vi "氨氮总磷平行样流程.vi"(9 "总磷1":bool, 10 "氨氮1":bool, 11 "队列输入":refnum<queue>) -> (3 "布尔":bool)   [LabVIEW 2016, in "质控单元.lvlib"]
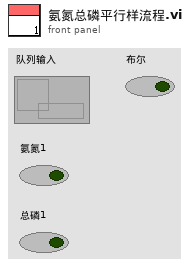
[diagram p1: front panel]
types:
  T1 = enum16{"待机", "启动氨氮水样", "氨氮测量中", "启动氨氮加标", "启动氨氮加标回收", "氨氮加标回收测量中", "启动总磷水样", "总磷水样测量中", "启动总磷加标", "启动总磷加标回收", "总磷加标回收测量中", "结束"}
  T2 = cluster{"站号":u16, "量程切换":enum32{"H", "L", "AUTO"}, "控制命令":enum16{"启动测量", "标样核查", "零点核查", "跨度核查", "空白测试", "平行样测试", "加标回收", "空白校准", "标样校准", "初始化（清洗）", "停止测试", "仪器重启", "校时", "模式设置", "测量间隔设置", "盲样测试"}, "模式设置":enum16{"待机", "连续模式", "周期模式", "定点模式", "受控模式", "手动模式"}, "测量间隔":u16}
  T3 = cluster{"时间标识":timestamp, "设备":string, "日志信息":string}
  T4 = cluster{"系统时间":timestamp, "工作状态":enum16{"空闲", "水样测试", "标样核查", "零点核查", "跨度核查", "空白测试", "平行样测试", "加标回收", "空白校准", "标样校准", "初始化（清洗）"}, "测量模式":enum16{"待机", "连续模式", "周期模式", "定点模式", "受控模式", "手动模式"}, "告警代码":u16, "故障代码":u16, "日志代码":u16, "软件版本":u16, "F0":sgl, "F1":sgl, "F2":sgl, "F3":sgl, "T":sgl, "H":sgl, "id":u16, "flowid":u16, "量程":u16, "总磷控温温度1":sgl, "营养盐控温温度2":sgl, "ADC":sgl}
  T5 = enum16{"空闲", "水样测试", "标样核查", "零点核查", "跨度核查", "空白测试", "平行样测试", "加标回收", "空白校准", "标样校准", "初始化（清洗）"}
  T6 = cluster{"因子编码":u32, "单位":u16, "标样参考值":sgl, "水样数据时间":timestamp, "水样实测值":sgl, "水样数据标识":string, "标样数据时间":timestamp, "标样实测值":sgl, "标样数据标识":string, "空白数据时间":timestamp, "空白实测值":sgl, "空白数据标识":string, "零点核查数据时间":timestamp, "零点核查实测值":sgl, "零点核查数据标识":string, "跨度核查数据时间":timestamp, "跨度核查实测值":sgl, "跨度核查数据标识":string, "加标回收数据时间":timestamp, "加标回收实测值":sgl, "加标回收数据标识":string, "平行样数据时间":timestamp, "平行样实测值":sgl, "平行样数据标识":string, "F0":sgl, "F1":sgl, "F2":sgl, "F3":sgl, "F4":sgl, "F5":sgl, "F6":sgl, "F7":sgl, "温度":sgl, "湿度":sgl, "X值":sgl, "fidrange":u16}
  T7 = cluster{"量程":dbl, "检出限":dbl, "加标前水样浓度":dbl, "加标后水样浓度":dbl, "加标水杯定容体积":dbl, "加标母液浓度":dbl, "加标体积":dbl, "加标回收率":dbl}
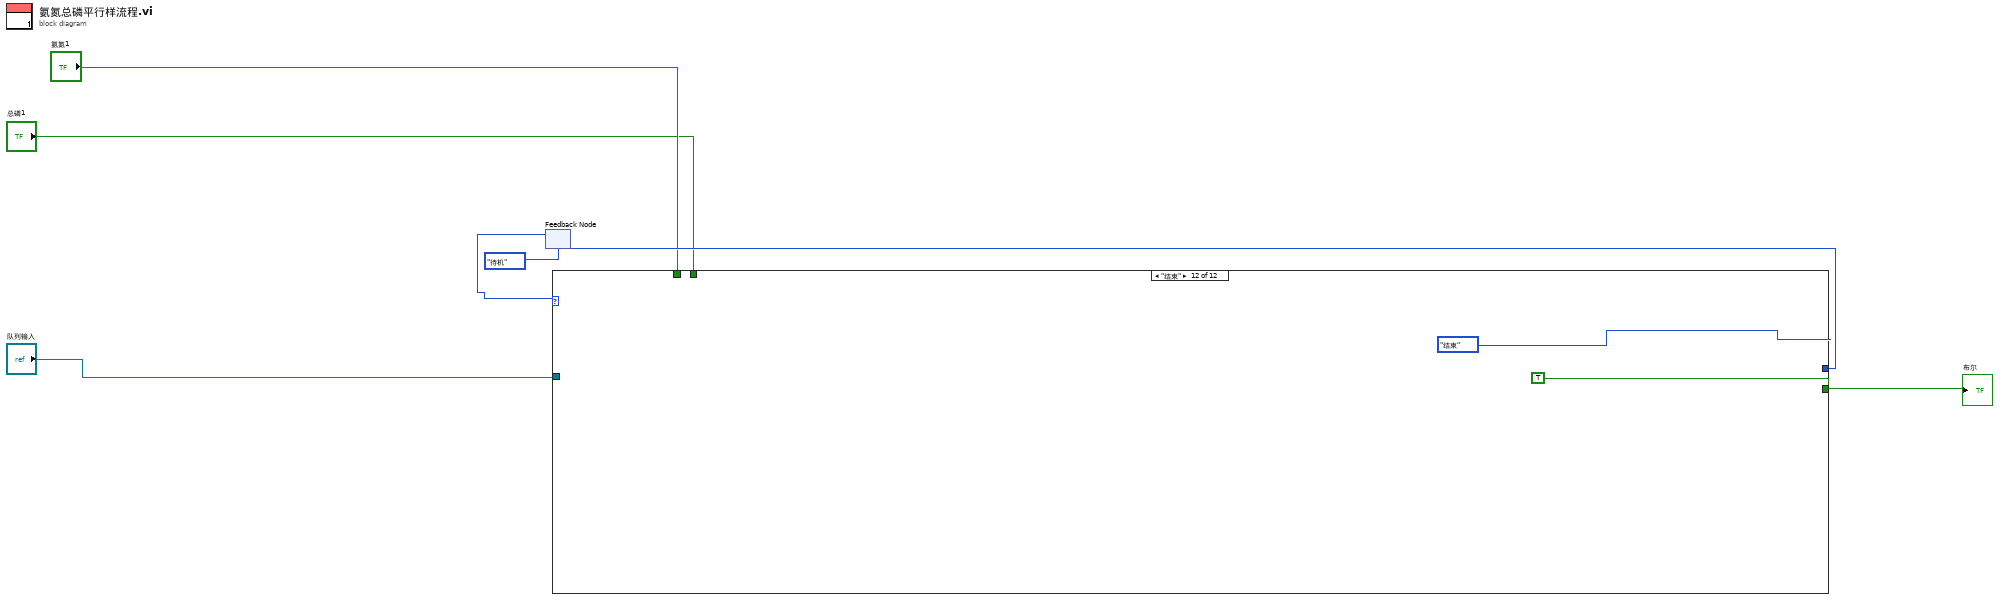
[diagram p0: block diagram]
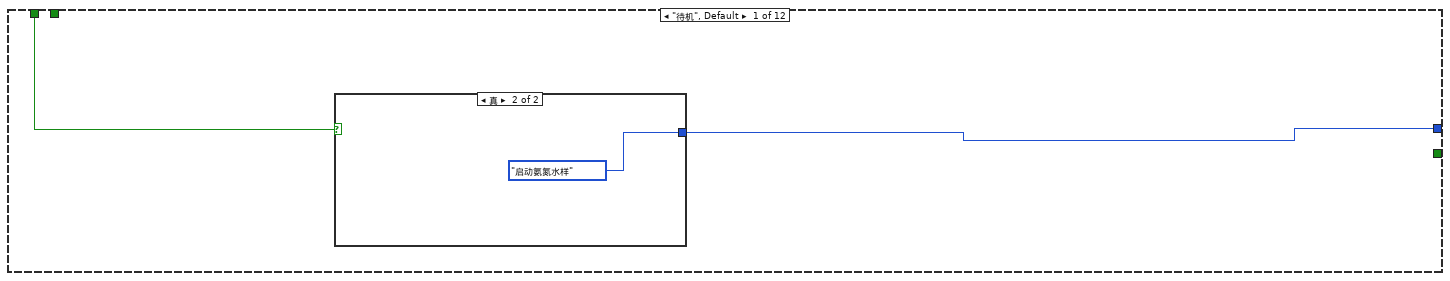
[diagram p2: hidden frame]
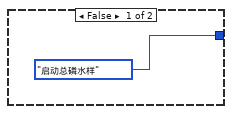
[diagram p3: hidden frame]
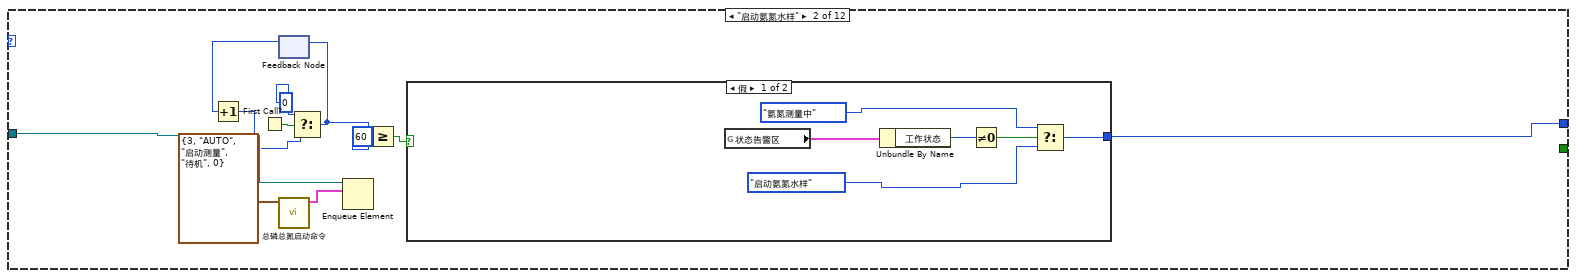
[diagram p4: hidden frame]
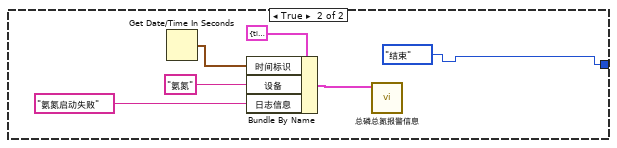
[diagram p5: hidden frame]
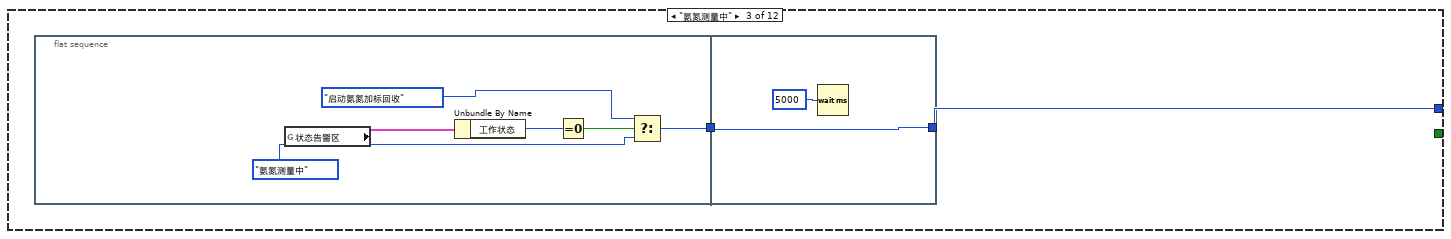
[diagram p6: hidden frame]
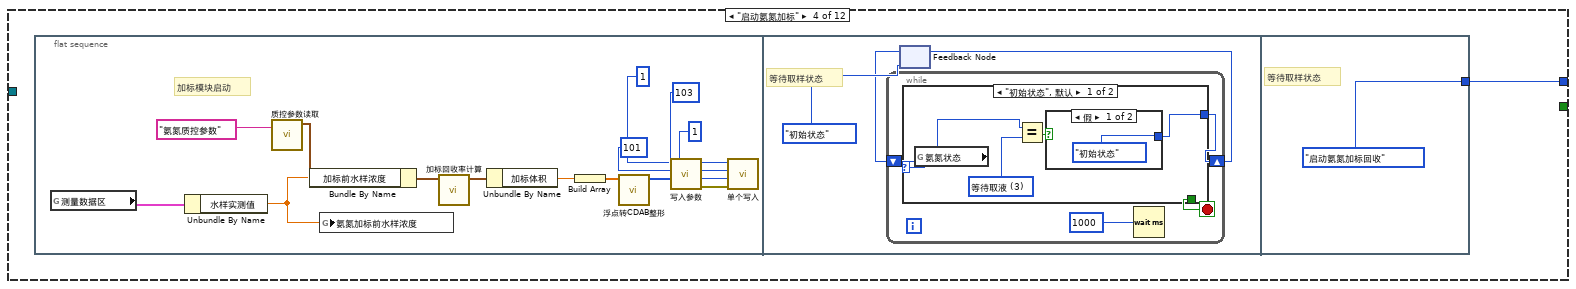
[diagram p7: hidden frame]
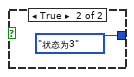
[diagram p8: hidden frame]
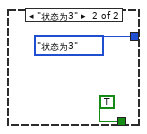
[diagram p9: hidden frame]
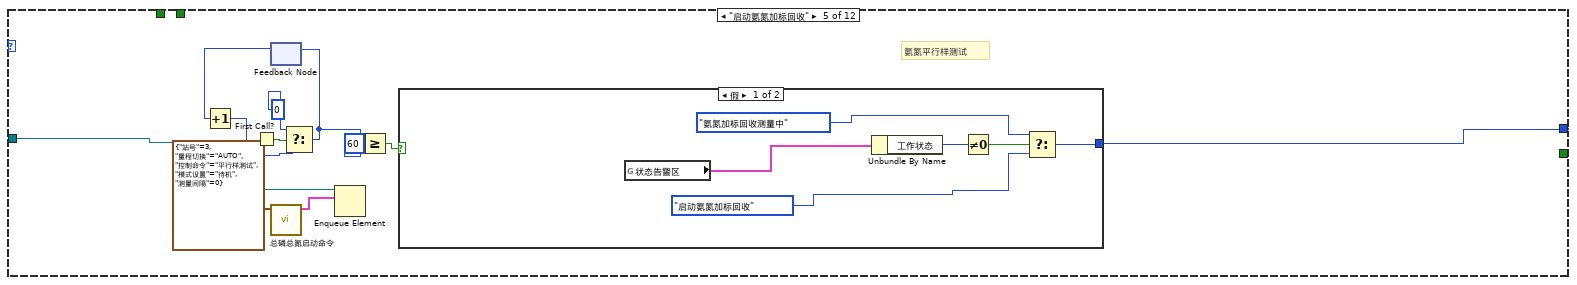
[diagram p10: hidden frame]
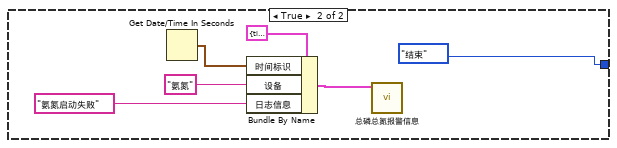
[diagram p11: hidden frame]
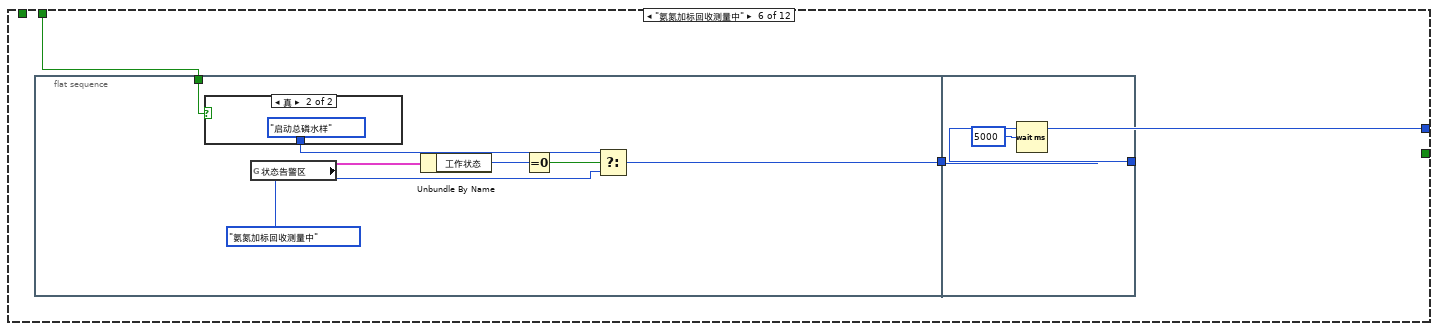
[diagram p12: hidden frame]
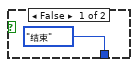
[diagram p13: hidden frame]
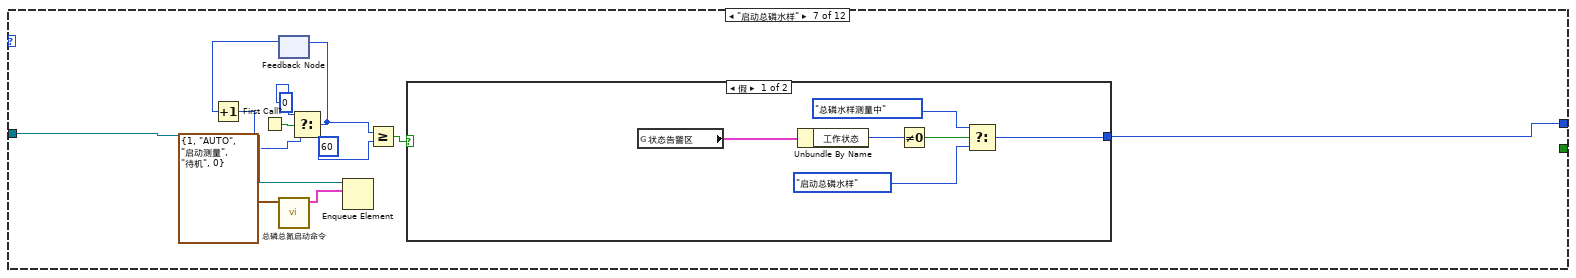
[diagram p14: hidden frame]
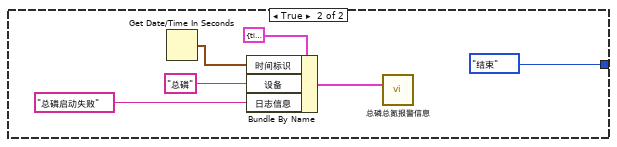
[diagram p15: hidden frame]
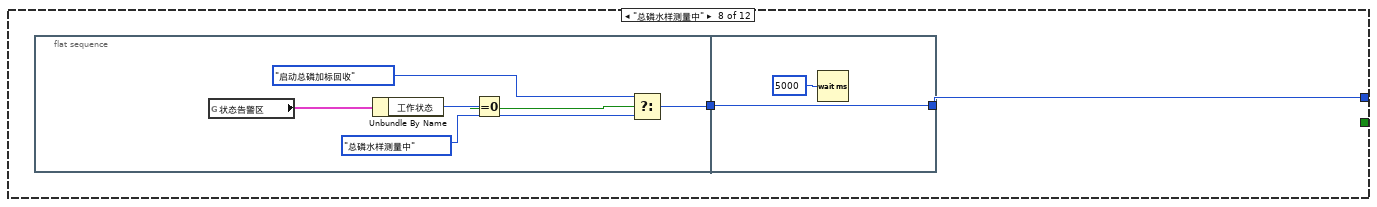
[diagram p16: hidden frame]
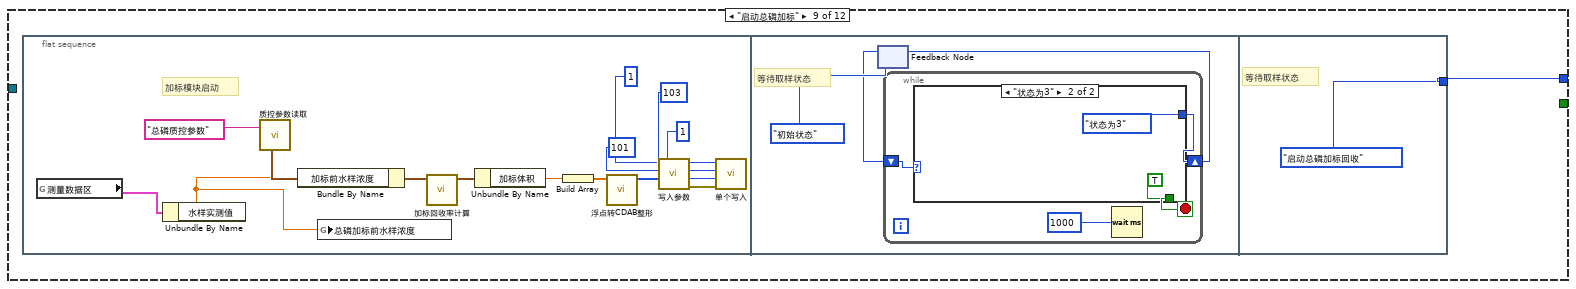
[diagram p17: hidden frame]
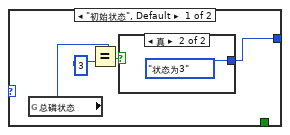
[diagram p18: hidden frame]
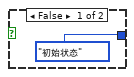
[diagram p19: hidden frame]
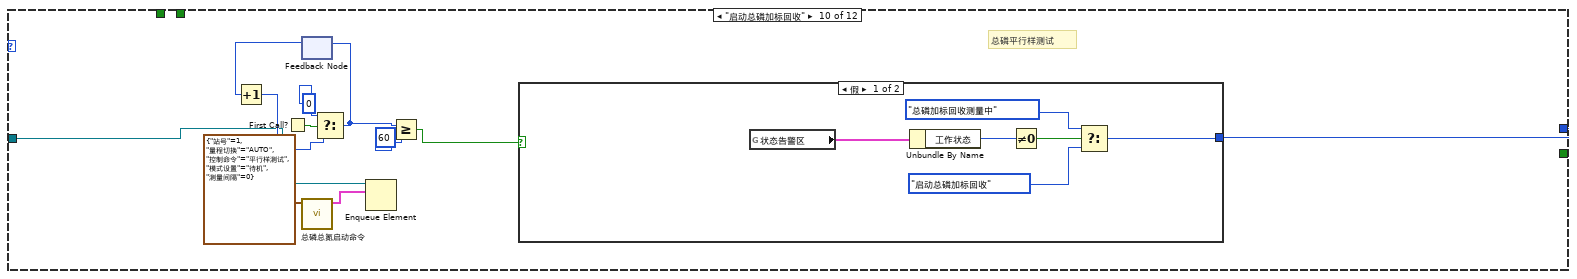
[diagram p20: hidden frame]
diagram:
  n1 = feedback #1(T1."待机") -> (w6:T1)
  n2 = case shown="\"结束\"" w6 {
    tunnel: [w8 w21 w36 w45 w76 w100 w122 w137 w146 w177 w200 T1."结束"] -> w5
    tunnel: "队列输入" -> [_ w22 _ _ w77 _ w123 _ _ w178 _ _]
    tunnel: [_ _ _ _ _ _ _ _ _ _ _ TRUE] -> w2
    tunnel: "总磷1" -> [_ _ _ _ _ w99 _ _ _ _ _ _]
    tunnel: "氨氮1" -> [w9 _ _ _ _ _ _ _ _ _ _ _]
    frame "待机", Default {
      n3 = case shown="真" w9 {
        tunnel: [T1."启动总磷水样" T1."启动氨氮水样"] -> w8
        frame False {
        }
        frame True {
        }
      }
    }
    frame "启动氨氮水样" {
      n4 = First Call?() -> (First Call?: T/F=w19:bool)
      n5 = feedback #2() -> (w18:i32)  [unwired: 1 in]
      n6 = Increment(x=w18) -> (x+1=w17:i32)
      n7 = call "总磷总氮启动命令.vi"("参数"=T2 {"站号"=3, "量程切换"=enum."AUTO", "控制命令"=enum."启动测量", "模式设置"=enum."待机", "测量间隔"=0}) -> ("启动命令"=w13:cluster{"命令":string, "data":variant})  [unwired: 10 in]
      n8 = Select(t=0, s=w19, f=w17) -> (s? t:f=w16:i32)
      n9 = feedback-in #2(w16) -> ()
      n10 = Enqueue Element(queue=w22, element=w13) -> ()  [unwired: 2 in, 3 out]
      n11 = Greater Or Equal?(x=w16, y=60) -> (x >= y?=w14:bool)
      n12 = case shown="假" w14 {
        tunnel: [w25 T1."结束"] -> w21
        frame False {
          n13 = global read "VAR总磷总氮全局变量.vi" "状态告警区"() -> (w28:T4)
          n14 = Unbundle By Name(w28) -> ("工作状态"=w27:T5)
          n15 = Not Equal To 0?(x=w27) -> (x != 0?=w26:bool)
          n16 = Select(t=T1."氨氮测量中", s=w26, f=T1."启动氨氮水样") -> (s? t:f=w25:T1)
        }
        frame True {
          n17 = Get Date/Time In Seconds() -> (seconds since 1Jan1904=w34:timestamp)
          n18 = Bundle By Name(cluster=T3 {"时间标识"=timestamp(0 s since 1904-01-01), "设备"="", "日志信息"=""} ("data in"), "时间标识"=w34, "设备"="氨氮", "日志信息"="氨氮启动失败") -> (w30:T3)
          n19 = call "总磷总氮报警信息.vi"("data in"=w30) -> ()  [unwired: 10 in, 1 out]
        }
      }
    }
    frame "氨氮测量中" {
      n20 = flat-sequence {
        tunnel: [w40] -> w35
        tunnel: [w44] -> w36
        tunnel: w35 -> [w44]
        frame #0 {
          n21 = global read "VAR总磷总氮全局变量.vi" "状态告警区"() -> (w41:T4)
          n22 = Unbundle By Name(w41) -> ("工作状态"=w42:T5)
          n23 = Equal To 0?(x=w42) -> (x = 0?=w39:bool)
          n24 = Select(t=T1."启动氨氮加标回收", s=w39, f=T1."氨氮测量中") -> (s? t:f=w40:T1)
        }
        frame #1 {
          n25 = Wait (ms)(milliseconds to wait=u32 5000 ("等待时间（毫秒）")) -> ()  [unwired: 1 out]
        }
      }
    }
    frame "启动氨氮加标" {
      n26 = flat-sequence {
        tunnel: [T1."启动氨氮加标回收"] -> w45
        frame #0 {
          w49 = u16 1 ("value")
          # "加标模块启动"
          n27 = global read "VAR总磷总氮全局变量.vi" "测量数据区"() -> (w47:T6)
          n28 = Unbundle By Name(w47) -> ("水样实测值"=w46:sgl)
          n29 = call "质控参数读取.vi"("section"="氨氮质控参数") -> ("参数"=w57:T7)  [unwired: 9 in, 1 out]
          n30 = Bundle By Name(cluster=w57, "加标前水样浓度"=w46) -> (w58:T7)
          n31 = global write "水样浓度全局.vi" "氨氮加标前水样浓度"(w46) -> ()
          n32 = call "加标回收率计算.vi"("参数"=w58) -> ("参数 out"=w56:T7)  [unwired: 10 in]
          n33 = Unbundle By Name(w56) -> ("加标体积"=w48:dbl)
          n34 = Build Array(w48) -> (w55:dbl[])
          n35 = call "浮点转CDAB整形.vi"("浮点数"=w55) -> ("CDAB整形输出"=w50:u16[])  [unwired: 10 in]
          n36 = call "写入参数.vi"("values"=w50, "starting address"=u16 101, "Slave ID"=w49) -> ("error out"=w54:errorcluster)  [unwired: 8 in]
          n37 = call "单个写入.vi"("Error in"=w54, "value"=u16 1, "address"=u16 103, "Slave ID"=w49) -> ()  [unwired: 7 in, 1 out]
        }
        frame #1 {
          # "等待取样状态"
          n38 = feedback #3(enum16{"初始状态", "状态为3"}."初始状态") -> (w61:enum16{"初始状态", "状态为3"})
          n39 = while {
            shift-right: [w65] -> w60
            shift-left: w61 -> [w66]
            stop <- w64 stop-if-true
            n40 = case shown="\"初始状态\", 默认" w66 {
              tunnel: [w68 enum16{"初始状态", "状态为3"}."状态为3"] -> w65
              tunnel: [_ TRUE] -> w64
              frame "初始状态", Default {
                w67 = u16 3 items=["待机", "润洗", "进样", "等待取液", "排液"] ("氨氮状态")
                n41 = global read "氨氮加标回收状态全局变量.vi" "氨氮状态"() -> (w70:u16)
                n42 = Equal?(x=w70, y=w67) -> (x = y?=w69:bool)
                n43 = case shown="假" w69 {
                  tunnel: [enum16{"初始状态", "状态为3"}."初始状态" enum16{"初始状态", "状态为3"}."状态为3"] -> w68
                  frame False {
                  }
                  frame True {
                  }
                }
              }
              frame "状态为3" {
              }
            }
            n44 = Wait (ms)(milliseconds to wait=u32 1000 ("等待时间（毫秒）")) -> ()  [unwired: 1 out]
          }
          n45 = feedback-in #3(w60) -> ()
        }
        frame #2 {
          # "等待取样状态"
        }
      }
    }
    frame "启动氨氮加标回收" {
      # "氨氮平行样测试"
      n46 = First Call?() -> (First Call?: T/F=w85:bool)
      n47 = feedback #4() -> (w84:i32)  [unwired: 1 in]
      n48 = Increment(x=w84) -> (x+1=w83:i32)
      n49 = call "总磷总氮启动命令.vi"("参数"=T2 {"站号"=3, "量程切换"=enum."AUTO", "控制命令"=enum."平行样测试", "模式设置"=enum."待机", "测量间隔"=0}) -> ("启动命令"=w79:cluster{"命令":string, "data":variant})  [unwired: 10 in]
      n50 = Select(t=0, s=w85, f=w83) -> (s? t:f=w82:i32)
      n51 = feedback-in #4(w82) -> ()
      n52 = Enqueue Element(queue=w77, element=w79) -> ()  [unwired: 2 in, 3 out]
      n53 = Greater Or Equal?(x=w82, y=60) -> (x >= y?=w80:bool)
      n54 = case shown="假" w80 {
        tunnel: [w89 T1."结束"] -> w76
        frame False {
          n55 = global read "VAR总磷总氮全局变量.vi" "状态告警区"() -> (w92:T4)
          n56 = Unbundle By Name(w92) -> ("工作状态"=w91:T5)
          n57 = Not Equal To 0?(x=w91) -> (x != 0?=w90:bool)
          n58 = Select(t=T1."氨氮加标回收测量中", s=w90, f=T1."启动氨氮加标回收") -> (s? t:f=w89:T1)
        }
        frame True {
          n59 = Get Date/Time In Seconds() -> (seconds since 1Jan1904=w98:timestamp)
          n60 = Bundle By Name(cluster=T3 {"时间标识"=timestamp(0 s since 1904-01-01), "设备"="", "日志信息"=""} ("data in"), "时间标识"=w98, "设备"="氨氮", "日志信息"="氨氮启动失败") -> (w94:T3)
          n61 = call "总磷总氮报警信息.vi"("data in"=w94) -> ()  [unwired: 10 in, 1 out]
        }
      }
    }
    frame "氨氮加标回收测量中" {
      n62 = flat-sequence {
        tunnel: [w106] -> w101
        tunnel: w99 -> [w102]
        tunnel: [w112] -> w100
        tunnel: w101 -> [w112]
        frame #0 {
          n63 = case shown="真" w102 {
            tunnel: [T1."结束" T1."启动总磷水样"] -> w104
            frame False {
            }
            frame True {
            }
          }
          n64 = global read "VAR总磷总氮全局变量.vi" "状态告警区"() -> (w107:T4)
          n65 = Unbundle By Name(w107) -> ("工作状态"=w108:T5)
          n66 = Equal To 0?(x=w108) -> (x = 0?=w103:bool)
          n67 = Select(t=w104, s=w103, f=T1."氨氮加标回收测量中") -> (s? t:f=w106:T1)
        }
        frame #1 {
          n68 = Wait (ms)(milliseconds to wait=u32 5000 ("等待时间（毫秒）")) -> ()  [unwired: 1 out]
        }
      }
    }
    frame "启动总磷水样" {
      n69 = First Call?() -> (First Call?: T/F=w120:bool)
      n70 = feedback #5() -> (w119:i32)  [unwired: 1 in]
      n71 = Increment(x=w119) -> (x+1=w118:i32)
      n72 = call "总磷总氮启动命令.vi"("参数"=T2 {"站号"=1, "量程切换"=enum."AUTO", "控制命令"=enum."启动测量", "模式设置"=enum."待机", "测量间隔"=0}) -> ("启动命令"=w114:cluster{"命令":string, "data":variant})  [unwired: 10 in]
      n73 = Select(t=0, s=w120, f=w118) -> (s? t:f=w117:i32)
      n74 = feedback-in #5(w117) -> ()
      n75 = Enqueue Element(queue=w123, element=w114) -> ()  [unwired: 2 in, 3 out]
      n76 = Greater Or Equal?(x=w117, y=60) -> (x >= y?=w115:bool)
      n77 = case shown="假" w115 {
        tunnel: [w126 T1."结束"] -> w122
        frame False {
          n78 = global read "VAR总磷总氮全局变量.vi" "状态告警区"() -> (w127:T4)
          n79 = Unbundle By Name(w127) -> ("工作状态"=w128:T5)
          n80 = Not Equal To 0?(x=w128) -> (x != 0?=w129:bool)
          n81 = Select(t=T1."总磷水样测量中", s=w129, f=T1."启动总磷水样") -> (s? t:f=w126:T1)
        }
        frame True {
          n82 = Get Date/Time In Seconds() -> (seconds since 1Jan1904=w135:timestamp)
          n83 = Bundle By Name(cluster=T3 {"时间标识"=timestamp(0 s since 1904-01-01), "设备"="", "日志信息"=""} ("data in"), "时间标识"=w135, "设备"="总磷", "日志信息"="总磷启动失败") -> (w131:T3)
          n84 = call "总磷总氮报警信息.vi"("data in"=w131) -> ()  [unwired: 10 in, 1 out]
        }
      }
    }
    frame "总磷水样测量中" {
      n85 = flat-sequence {
        tunnel: [w141] -> w136
        tunnel: [w145] -> w137
        tunnel: w136 -> [w145]
        frame #0 {
          n86 = global read "VAR总磷总氮全局变量.vi" "状态告警区"() -> (w142:T4)
          n87 = Unbundle By Name(w142) -> ("工作状态"=w143:T5)
          n88 = Equal To 0?(x=w143) -> (x = 0?=w140:bool)
          n89 = Select(t=T1."启动总磷加标回收", s=w140, f=T1."总磷水样测量中") -> (s? t:f=w141:T1)
        }
        frame #1 {
          n90 = Wait (ms)(milliseconds to wait=u32 5000 ("等待时间（毫秒）")) -> ()  [unwired: 1 out]
        }
      }
    }
    frame "启动总磷加标" {
      n91 = flat-sequence {
        tunnel: [T1."启动总磷加标回收"] -> w146
        frame #0 {
          w151 = u16 1 ("value")
          # "加标模块启动"
          n92 = global read "VAR总磷总氮全局变量.vi" "测量数据区"() -> (w149:T6)
          n93 = Unbundle By Name(w149) -> ("水样实测值"=w147:sgl)
          n94 = call "质控参数读取.vi"("section"="总磷质控参数") -> ("参数"=w148:T7)  [unwired: 9 in, 1 out]
          n95 = Bundle By Name(cluster=w148, "加标前水样浓度"=w147) -> (w159:T7)
          n96 = global write "水样浓度全局.vi" "总磷加标前水样浓度"(w147) -> ()
          n97 = call "加标回收率计算.vi"("参数"=w159) -> ("参数 out"=w158:T7)  [unwired: 10 in]
          n98 = Unbundle By Name(w158) -> ("加标体积"=w150:dbl)
          n99 = Build Array(w150) -> (w157:dbl[])
          n100 = call "浮点转CDAB整形.vi"("浮点数"=w157) -> ("CDAB整形输出"=w152:u16[])  [unwired: 10 in]
          n101 = call "写入参数.vi"("values"=w152, "starting address"=u16 101, "Slave ID"=w151) -> ("error out"=w156:errorcluster)  [unwired: 8 in]
          n102 = call "单个写入.vi"("Error in"=w156, "value"=u16 1, "address"=u16 103, "Slave ID"=w151) -> ()  [unwired: 7 in, 1 out]
        }
        frame #1 {
          # "等待取样状态"
          n103 = feedback #6(enum16{"初始状态", "状态为3"}."初始状态") -> (w162:enum16{"初始状态", "状态为3"})
          n104 = while {
            shift-right: [w166] -> w161
            shift-left: w162 -> [w167]
            stop <- w165 stop-if-true
            n105 = case shown="\"状态为3\"" w167 {
              tunnel: [w168 enum16{"初始状态", "状态为3"}."状态为3"] -> w166
              tunnel: [_ TRUE] -> w165
              frame "初始状态", Default {
                n106 = global read "氨氮加标回收状态全局变量.vi" "总磷状态"() -> (w170:u16)
                n107 = Equal?(x=w170, y=u16 3) -> (x = y?=w169:bool)
                n108 = case shown="真" w169 {
                  tunnel: [enum16{"初始状态", "状态为3"}."初始状态" enum16{"初始状态", "状态为3"}."状态为3"] -> w168
                  frame False {
                  }
                  frame True {
                  }
                }
              }
              frame "状态为3" {
              }
            }
            n109 = Wait (ms)(milliseconds to wait=u32 1000 ("等待时间（毫秒）")) -> ()  [unwired: 1 out]
          }
          n110 = feedback-in #6(w161) -> ()
        }
        frame #2 {
          # "等待取样状态"
        }
      }
    }
    frame "启动总磷加标回收" {
      # "总磷平行样测试"
      n111 = First Call?() -> (First Call?: T/F=w186:bool)
      n112 = feedback #7() -> (w185:i32)  [unwired: 1 in]
      n113 = Increment(x=w185) -> (x+1=w184:i32)
      n114 = call "总磷总氮启动命令.vi"("参数"=T2 {"站号"=1, "量程切换"=enum."AUTO", "控制命令"=enum."平行样测试", "模式设置"=enum."待机", "测量间隔"=0}) -> ("启动命令"=w180:cluster{"命令":string, "data":variant})  [unwired: 10 in]
      n115 = Select(t=0, s=w186, f=w184) -> (s? t:f=w183:i32)
      n116 = feedback-in #7(w183) -> ()
      n117 = Enqueue Element(queue=w178, element=w180) -> ()  [unwired: 2 in, 3 out]
      n118 = Greater Or Equal?(x=w183, y=60) -> (x >= y?=w181:bool)
      n119 = case shown="假" w181 {
        tunnel: [w190 T1."结束"] -> w177
        frame False {
          n120 = global read "VAR总磷总氮全局变量.vi" "状态告警区"() -> (w191:T4)
          n121 = Unbundle By Name(w191) -> ("工作状态"=w192:T5)
          n122 = Not Equal To 0?(x=w192) -> (x != 0?=w193:bool)
          n123 = Select(t=T1."总磷加标回收测量中", s=w193, f=T1."启动总磷加标回收") -> (s? t:f=w190:T1)
        }
        frame True {
          n124 = Get Date/Time In Seconds() -> (seconds since 1Jan1904=w199:timestamp)
          n125 = Bundle By Name(cluster=T3 {"时间标识"=timestamp(0 s since 1904-01-01), "设备"="", "日志信息"=""} ("data in"), "时间标识"=w199, "设备"="总磷", "日志信息"="总磷启动失败") -> (w195:T3)
          n126 = call "总磷总氮报警信息.vi"("data in"=w195) -> ()  [unwired: 10 in, 1 out]
        }
      }
    }
    frame "总磷加标回收测量中" {
      n127 = flat-sequence {
        tunnel: [w205] -> w201
        tunnel: [w209] -> w200
        tunnel: w201 -> [w209]
        frame #0 {
          n128 = global read "VAR总磷总氮全局变量.vi" "状态告警区"() -> (w206:T4)
          n129 = Unbundle By Name(w206) -> ("工作状态"=w207:T5)
          n130 = Equal To 0?(x=w207) -> (x = 0?=w202:bool)
          n131 = Select(t=T1."结束", s=w202, f=T1."总磷加标回收测量中") -> (s? t:f=w205:T1)
        }
        frame #1 {
          n132 = Wait (ms)(milliseconds to wait=u32 5000 ("等待时间（毫秒）")) -> ()  [unwired: 1 out]
        }
      }
    }
    frame "结束" {
    }
  }
  "布尔" <- w2
  n133 = feedback-in #1(w5) -> ()
